vi "Requests.vi"(8 "error in (no error)":errorcluster, 9 "write enable":bool=TRUE, 11 "LIR-919 in":refnum<class "LIR-919D.lvclass">) -> (0 "error out":errorcluster, 3 "LIR-919 out":refnum<class "LIR-919D.lvclass">)   [LabVIEW 2021, in "LIR-919D.lvclass"]
uses:
  LIR-919D.lvclass
  D:/my_projects/projects/Algorithms/Labview/21/Modbus_v121c/Network Protocol/MB/Modbus Master CR.lvclass
  D:/my_projects/projects/Algorithms/Labview/21/Modbus_v121c/Network Protocol/Network Master/Network Master.lvclass
  Modbus Master CR.lvclass/Modbus Master CR.ctl
  Modbus Data Unit/Modbus Data Unit.lvclass/Modbus Data Unit.ctl
  Network Master/Network Master.lvclass/Network Master.ctl
  Master Function Definition/Write Multiple Registers Request.vi
  Master Function Definition/Function data mismatch error.vi
  Master Function Definition/Write Multiple Registers Response.vi
  Network Master/Read write Master.vi
  Master Function Definition/Read Input Registers Request.vi
  Master Function Definition/Read Input Registers Response.vi
  Master Function Definition/Read Holding Registers Request.vi
  Master Function Definition/Read Holding Registers Response.vi
  Modbus Data Unit/Construct PDU.vi
  Utility/U16s to Bytes.vi
  Master Function Definition/Function code mismatch error.vi
  Data Model/Error Generator.vi
  Modbus Data Unit/Deconstruct PDU.vi
  Utility/Bytes to U16s.vi
  Modbus Data Unit/Modbus Data Unit.lvclass
  Data Model/Device Data Model.lvclass
  Transmission Data Unit/Transmission Data Unit.lvclass
  Modbus Master CR.lvclass
  Network Master/Network Master.lvclass
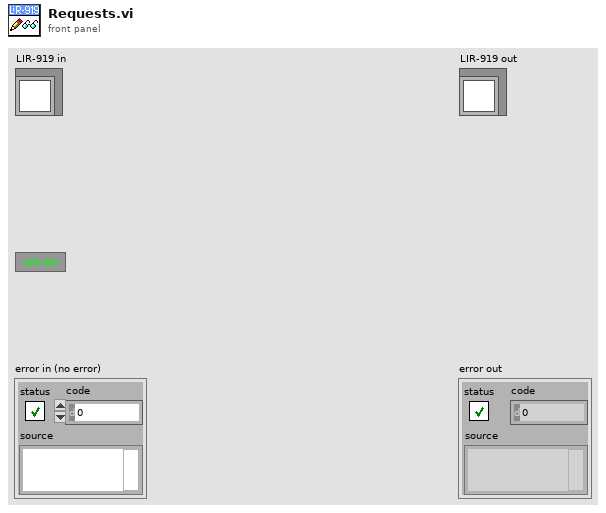
[diagram p1: front panel]
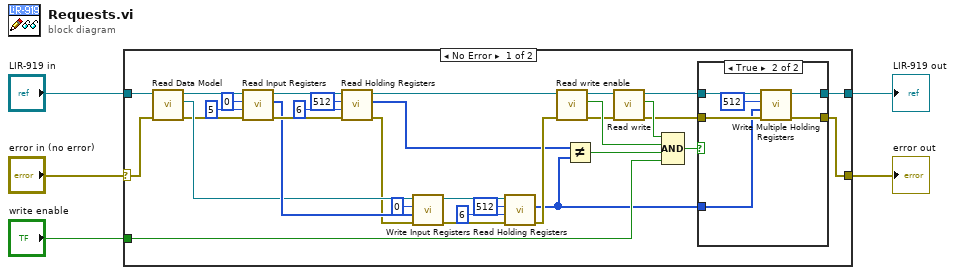
[diagram p0: block diagram]
diagram:
  n1 = case shown="No Error" "error in (no error)" {
    selector: "error in (no error)" -> [w7 w48]
    tunnel: [w36 w48] -> w3
    tunnel: [w11 w47] -> w4
    tunnel: "LIR-919 in" -> [w30 w47]
    tunnel: "write enable" -> [w15 _]
    frame No Error {
      n2 = call "Read Data Model.vi"("error in (no error)"=w7, "MB_TCP in"=w30) -> ("error out"=w6:errorcluster, "Data Model"=w29:refnum<class "Device Data Model.lvclass">, "MB_TCP out"=w28:refnum<class "LIR-919D.lvclass">)  [unwired: 7 in]
      n3 = call "Read Input Registers.vi"("error in (no error)"=w6, "number of input registers"=u16 5 ("number of discrete inputs"), "starting address"=u16 0, "Modbus master in"=w28) -> ("error out"=w34:errorcluster, "register values"=w31:u16[], "Modbus master out"=w35:refnum<class "LIR-919D.lvclass">)  [unwired: 5 in]
      n4 = call "Read Holding Registers.vi"("error in (no error)"=w34, "number of holding registers"=u16 6 ("number of discrete inputs"), "starting address"=u16 512, "Modbus master in"=w35) -> ("error out"=w27:errorcluster, "register values"=w9:u16[], "Modbus master out"=w17:refnum<class "LIR-919D.lvclass">)  [unwired: 5 in]
      n5 = call-dynamic "Write Input Registers.vi"("error in (no error)"=w27, "register values"=w31, "starting address"=u16 0, "Device Data Model in"=w29) -> ("error out"=w26:errorcluster, "Device Data Model out"=w25:refnum<class "Device Data Model.lvclass">)  [unwired: 6 in]
      n6 = call-dynamic "Read Holding Registers.vi"("error in"=w26, "number of registers"=u16 6 ("number of discrete inputs"), "starting address"=u16 512, "device data model in"=w25) -> ("error out"=w16:errorcluster, "data"=w10:u16[])  [unwired: 5 in, 1 out]
      n7 = call "Read write enable.vi"("error in (no error)"=w16, "MB in"=w17) -> ("error out"=w19:errorcluster, "write enable"=w21:bool, "MB out"=w20:refnum<class "LIR-919D.lvclass">)  [unwired: 7 in]
      n8 = Not Equal?(x=w9, y=w10) -> (x != y?=w22:bool)
      n9 = call "Read write.vi"("error in (no error)"=w19, "MB in"=w20) -> ("error out"=w13:errorcluster, "Write"=w18:bool, "MB out"=w12:refnum<class "LIR-919D.lvclass">)  [unwired: 7 in]
      n10 = Compound Arithmetic op=AND(w18, w21, w22, w15) -> (w14:bool)
      n11 = case shown="True" w14 {
        tunnel: w13 -> [w40 w45]
        tunnel: [w40 w43] -> w36
        tunnel: w12 -> [w39 w46]
        tunnel: w10 -> [_ w42]
        tunnel: [w39 w41] -> w11
        frame False {
        }
        frame True {
          n12 = call "Write Multiple Holding Registers.vi"("error in (no error)"=w45, "holding register values"=w42, "starting address"=u16 512, "Modbus master in"=w46) -> ("error out"=w43:errorcluster, "Modbus master out"=w41:refnum<class "LIR-919D.lvclass">)  [unwired: 6 in]
        }
      }
    }
    frame Error {
    }
  }
  "error out" <- w3
  "LIR-919 out" <- w4
